vi "Remove Panel by Index.vi"(8 "error in (no error)":errorcluster, 10 "Index":i32, 11 "PanelArray in":refnum<class "PanelArray.lvclass">) -> (0 "error out":errorcluster, 2 "Removed Panel":refnum<class "Panel.lvclass">, 3 "PanelArray out":refnum<class "PanelArray.lvclass">)   [LabVIEW 2018, in "OOPanel.lvlib" / "PanelArray.lvclass"]
uses:
  PanelArray.lvclass
  Panel/Panel.lvclass
  PanelArray.lvclass/PanelArray.ctl
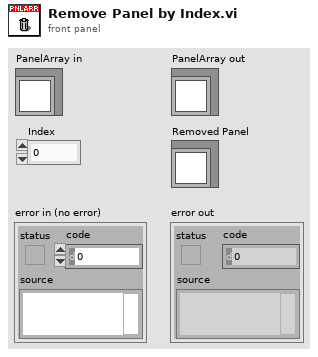
[diagram p1: front panel]
types:
  T1 = typedef "OOPanel.lvlib/PanelArray.lvclass/Ref Data.ctl" = cluster{"State":T2, "Refs":T3, "Events":T4, "Scrolling":T5, "Panels":T6}
  T2 = typedef "OOPanel.lvlib/PanelArray.lvclass/State.ctl" = cluster{"Defer Updates":bool, "Running":bool, "Dynamic Sizing":bool, "Borders":bool}
  T3 = typedef "OOPanel.lvlib/PanelArray.lvclass/Refs.ctl" = cluster{"SubPanels":refnum<vi>[], "Scrollbar":refnum<vi>, "Owning Panel":refnum<vi>}
  T4 = typedef "OOPanel.lvlib/PanelArray.lvclass/Events.ctl" = cluster{"Close":refnum<user-event>}
  T5 = typedef "OOPanel.lvlib/PanelArray.lvclass/Scrolling.ctl" = cluster{"Size":i32, "Max":i32, "Current":i32, "Top Index":i32, "Heights":i32[]}
  T6 = typedef "OOPanel.lvlib/PanelArray.lvclass/Panels.ctl" = cluster{"All":refnum<class "Panel.lvclass">[], "Visible":refnum<class "Panel.lvclass">[], "Blank":refnum<class "ArrayBlank.lvclass">}
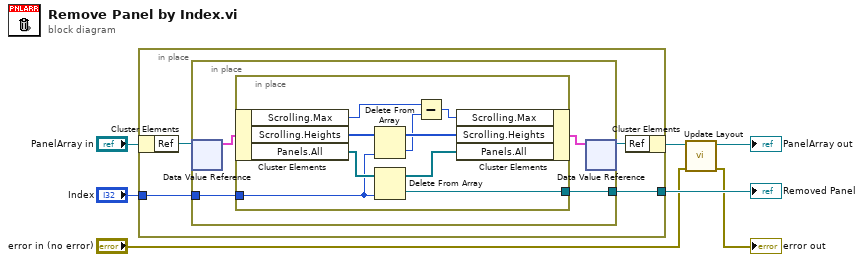
[diagram p0: block diagram]
diagram:
  n1 = in-place {
    in-place-border: "Index" -> [w11]
    in-place-border: [w10] -> w6
    n2 = in-place-cluster #1("PanelArray in") -> ("Ref"=w9:refnum<data-value>)
    n3 = in-place {
      in-place-border: w11 -> [w15]
      in-place-border: [w14] -> w10
      n4 = in-place-dvr #2(w9) -> (w13:T1)  [unwired: 1 out]
      n5 = in-place {
        in-place-border: w15 -> [w20]
        in-place-border: [w24] -> w14
        n6 = in-place-cluster #3(w13) -> ("Scrolling.Max"=w17:i32, "Scrolling.Heights"=w21:i32[], "Panels.All"=w23:refnum<class "Panel.lvclass">[])
        n7 = Delete From Array(array=w21, index=w20) -> (deleted portion=w18:i32, array with subset deleted=w19:i32[])  [unwired: 1 in]
        n8 = Delete From Array(array=w23, index=w20) -> (deleted portion=w24:refnum<class "Panel.lvclass">, array with subset deleted=w22:refnum<class "Panel.lvclass">[])  [unwired: 1 in]
        n9 = Subtract(x=w17, y=w18) -> (x-y=w16:i32)
        n10 = in-place-cluster #3("Scrolling.Max"=w16, "Scrolling.Heights"=w19, "Panels.All"=w22) -> (w12:T1)
      }
      n11 = in-place-dvr #2(w12) -> (w8:refnum<data-value>)  [unwired: 1 out]
    }
    n12 = in-place-cluster #1("Ref"=w8) -> (w4:refnum<class "PanelArray.lvclass">)
  }
  "Removed Panel" <- w6
  n13 = call "Update Layout.vi"("error in (no error)"="error in (no error)", "PanelArray in"=w4) -> ("error out"=→"error out":errorcluster, "PanelArray out"=→"PanelArray out":refnum<class "PanelArray.lvclass">)  [unwired: 8 in]
